vi "_Raise Document Title Changed.vi"(4 "WebView2.lvlib:WebView2 Control.lvclass":refnum<class "WebView2 Control.lvclass">, 5 "Event Data":cluster{"sender":refnum<k24>, "e":refnum<k24>}, 6 "Control Ref":refnum<k24>, 7 "Event Common Data":T1) -> ()   [LabVIEW 2020, in "WebView2.lvlib" / "WebView2 Control.lvclass"]
uses:
  WebView2 Control.lvclass
  C:/Users/Simon/Documents/GitHub/LV-WebView2/Source/Libs/Microsoft.Web.WebView2.Core.dll
  Libs/Microsoft.Web.WebView2.Core.dll
  WebView2 Control.lvclass/WebView2 Control.ctl
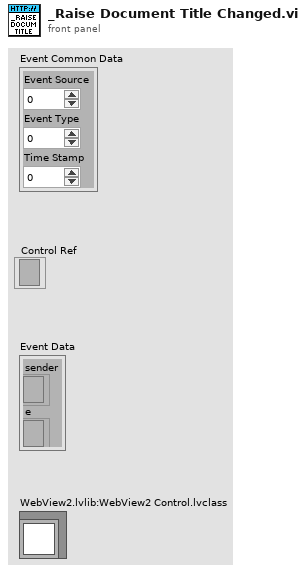
[diagram p1: front panel]
types:
  T1 = cluster{"Event Source":i32, "Event Type":u32, "Time Stamp":u32}
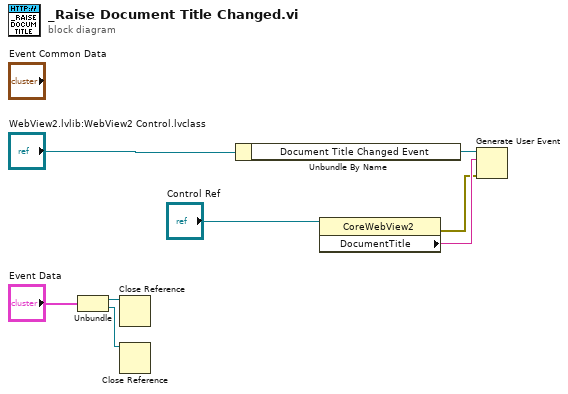
[diagram p0: block diagram]
diagram:
  n1 = Unbundle("Event Data") -> ("sender"=w2:refnum<k24>, "e"=w1:refnum<k24>)
  n2 = Close Reference(reference=w2) -> ()  [unwired: 1 in, 1 out]
  n3 = Close Reference(reference=w1) -> ()  [unwired: 1 in, 1 out]
  n4 = Unbundle By Name("WebView2.lvlib:WebView2 Control.lvclass") -> ("Document Title Changed Event"=w6:refnum<user-event>)
  n5 = property class="CoreWebView2"(reference="Control Ref") -> (error out=w4:errorcluster, "DocumentTitle"=w5:string)  [unwired: 1 in, 1 out]
  n6 = Generate User Event(user event=w6, event data cluster=w5, error in=w4) -> ()  [unwired: 1 in, 2 out]
